vi "IMU Initialization VI.vi"(8 "error in (no error)":errorcluster, 10 "Custom XML":string, 11 "Device Item Ref in":T1 format="%.0x") -> (0 "error out":errorcluster, 3 "Device Item Ref out":T1 format="%.0x")   [LabVIEW 2015, in "IMU Custom Device.lvlib"]
uses:
  IMU Custom Device.lvlib
  <vilib>/NI Veristand/Custom Device API/Custom Device Item Ref.ctl
  <vilib>/NI Veristand/Custom Device API/Custom Device Channel.ctl
  <vilib>/NI Veristand/Custom Device API/Custom Device Channel Type.ctl
  <vilib>/NI Veristand/Custom Device API/Custom Device API.lvlib
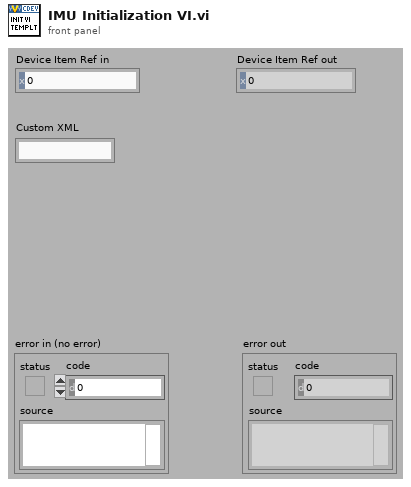
[diagram p1: front panel]
types:
  T1 = typedef "Custom Device API.lvlib/Custom Device Item Ref.ctl" = u64
  T2 = typedef "Custom Device API.lvlib/Custom Device Channel.ctl" = cluster{"Type":T3, "Units":string, "Default Value":dbl, "Faultable":bool, "Scalable":bool}
  T3 = typedef "Custom Device API.lvlib/Custom Device Channel Type.ctl" = enum16{"Input", "Output"}
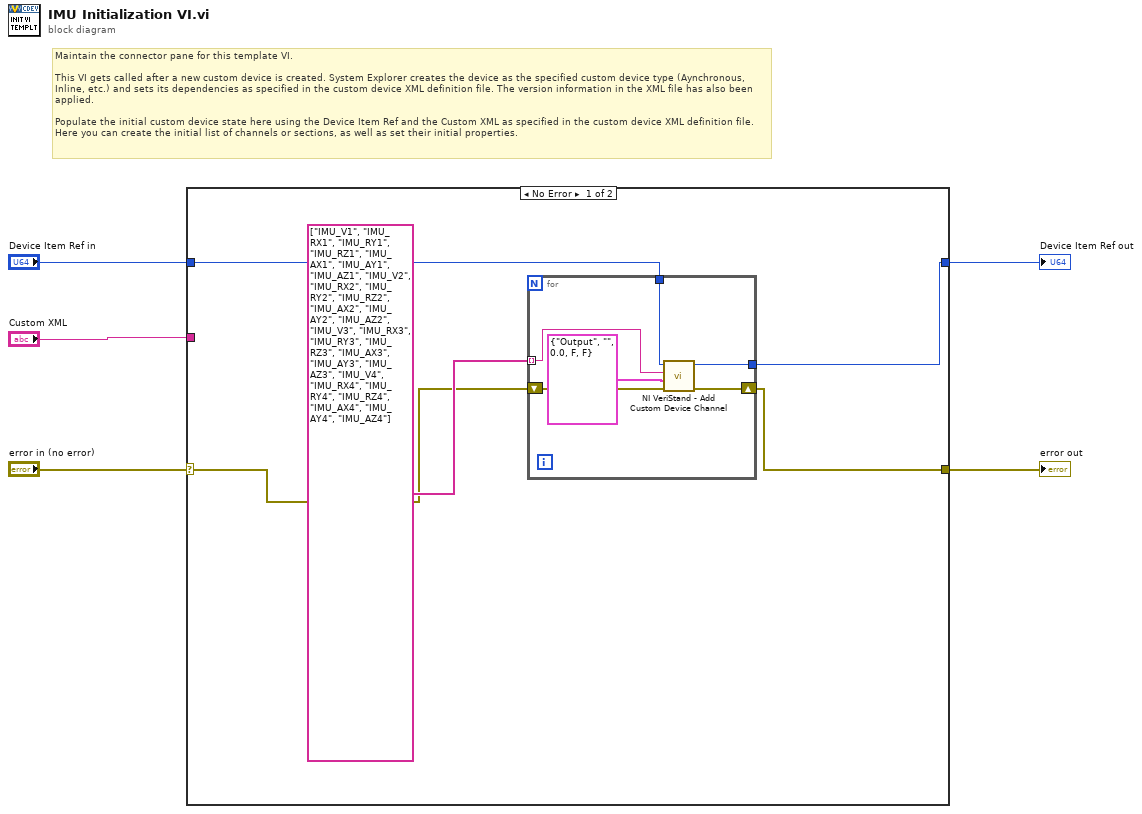
[diagram p0: block diagram]
diagram:
  # "Maintain the connector pane for this template VI.\n\nThis VI gets called after a new custom device is created. System Explorer creates the device as the specified custom device type (Aynchronous, Inline, etc.) and sets its dependencies as specified in the custom device XML definition file. The version information in the XML file has also been applied.\n\nPopulate the initial custom device state here using the Device Item Ref and the Custom XML as specified in the custom device XML definition file. Here you can create the initial list of channels or sections, as well as set their initial properties."
  n1 = case shown="No Error" "error in (no error)" {
    selector: "error in (no error)" -> [w7 w18]
    tunnel: [w6 w18] -> w1
    tunnel: [w8 w17] -> w2
    tunnel: "Device Item Ref in" -> [w9 w17]
    tunnel: "Custom XML" -> [_ _]
    frame No Error {
      n2 = for {
        tunnel: string[] ["IMU_V1", "IMU_RX1", "IMU_RY1", "IMU_RZ1", "IMU_AX1", "IMU_AY1", "IMU_AZ1", "IMU_V2", "IMU_RX2", "IMU_RY2", "IMU_RZ2", "IMU_AX2", "IMU_AY2", "IMU_AZ2", "IMU_V3", "IMU_RX3", "IMU_RY3", "IMU_RZ3", "IMU_AX3", "IMU_AY3", "IMU_AZ3", "IMU_V4", "IMU_RX4", "IMU_RY4", "IMU_RZ4", "IMU_AX4", "IMU_AY4", "IMU_AZ4"] -> [w16] mode=indexing
        tunnel: w9 -> [w14]
        tunnel: [w13] -> w8
        shift-right: [w11] -> w6
        shift-left: w7 -> [w12]
        n3 = call <vilib>:"NI VeriStand - Add Custom Device Channel.vi"("error in (no error)"=w12, "Channel"=T2 {"Type"=enum."Output", "Units"="", "Default Value"=0.0, "Faultable"=FALSE, "Scalable"=FALSE}, "Channel Name"=w16, "Parent Ref in"=w14) -> ("error out"=w11:errorcluster, "Parent Ref out"=w13:T1)  [unwired: 4 in, 2 out]
      }
    }
    frame Error {
    }
  }
  "error out" <- w1
  "Device Item Ref out" <- w2
